vi "Auto_Conf.vi"() -> ()   [LabVIEW 2015]
panel:
  in  "Auto3TrimmedCommand":string
  in  "Auto2CurrentCommand":string
  in  "Auto1FileStatus":string
  in  "Auto0CurrentFile":string
  in  "Has Turned":bool
  in  "AutoToRun":u8
  # "Integers"
  # "Booleans"
  # "Strings"
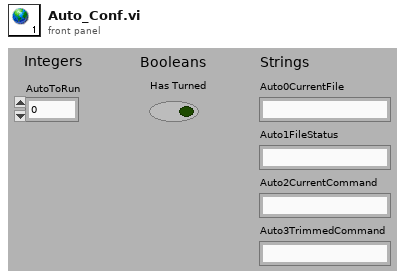
[diagram p1: front panel]
diagram:
